vi "Check Escala.vi"(8 "error in (no error)":errorcluster, 10 "Grandeza":string, 11 "189 in":refnum<class "189.lvclass">) -> (0 "error out":errorcluster, 2 "Escala Correta?":bool, 3 "189 out":refnum<class "189.lvclass">)   [LabVIEW 2015, in "189.lvclass"]
uses:
  189.lvclass
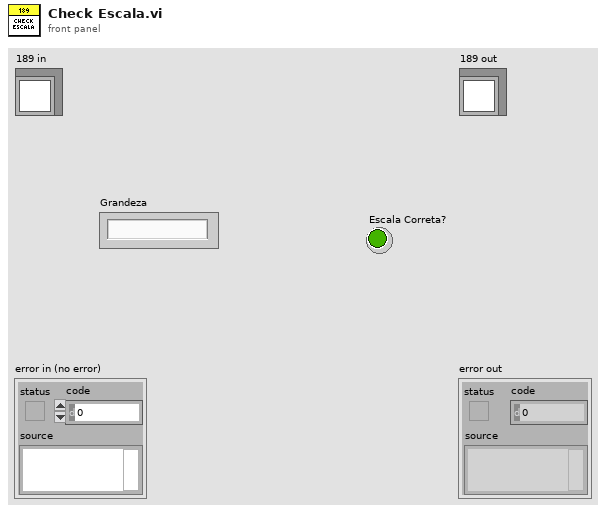
[diagram p1: front panel]
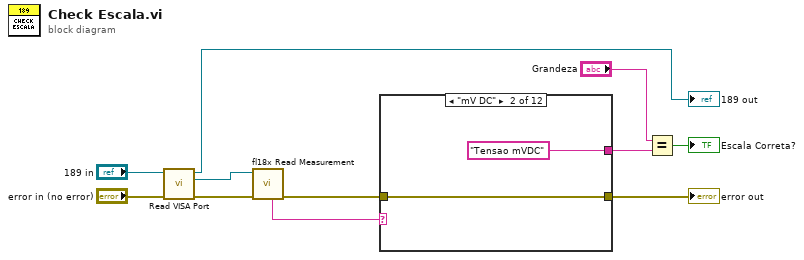
[diagram p0: block diagram]
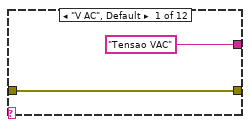
[diagram p2: hidden frame]
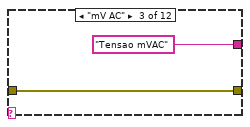
[diagram p3: hidden frame]
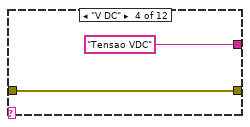
[diagram p4: hidden frame]
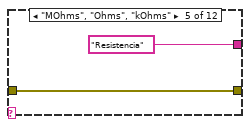
[diagram p5: hidden frame]
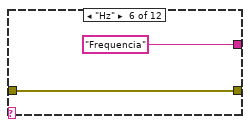
[diagram p6: hidden frame]
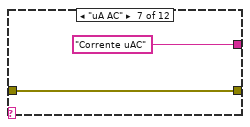
[diagram p7: hidden frame]
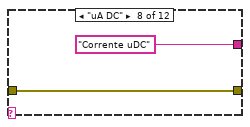
[diagram p8: hidden frame]
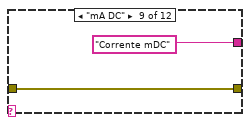
[diagram p9: hidden frame]
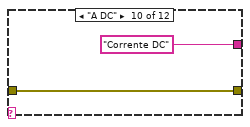
[diagram p10: hidden frame]
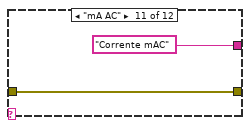
[diagram p11: hidden frame]
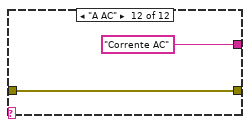
[diagram p12: hidden frame]
diagram:
  n1 = call-dynamic "Read VISA Port.vi"("error in (no error)"="error in (no error)", "Device in"="189 in") -> ("error out"=w8:errorcluster, "VISA Port"=w9:refnum<visa-resource-name>, "Device out"=→"189 out":refnum<class "189.lvclass">)  [unwired: 7 in]
  n2 = call <instrlib>:"fl18x Read Measurement.vi"("error in (no error)"=w8, "VISA session"=w9) -> ("error out"=w7:errorcluster, "Unidade"=w6:string)  [unwired: 5 in, 3 out]
  n3 = case shown="\"mV DC\"" w6 {
    tunnel: [w13 w15 w17 w19 w21 w23 w25 w27 w29 w31 w33 w35] -> w2
    tunnel: w7 -> [w13 w15 w17 w19 w21 w23 w25 w27 w29 w31 w33 w35]
    tunnel: ["Tensao VAC" "Tensao mVDC" "Tensao mVAC" "Tensao VDC" "Resistencia" "Frequencia" "Corrente uAC" "Corrente uDC" "Corrente mDC" "Corrente DC" "Corrente mAC" "Corrente AC"] -> w5
    frame "V AC", Default {
    }
    frame "mV DC" {
    }
    frame "mV AC" {
    }
    frame "V DC" {
    }
    frame "MOhms", "Ohms", "kOhms" {
    }
    frame "Hz" {
    }
    frame "uA AC" {
    }
    frame "uA DC" {
    }
    frame "mA DC" {
    }
    frame "A DC" {
    }
    frame "mA AC" {
    }
    frame "A AC" {
    }
  }
  "error out" <- w2
  n4 = Equal?(x="Grandeza", y=w5) -> (x = y?=→"Escala Correta?":bool)
